vi "Read Pulse Recorder Configuration.vi"(8 "error in (no error)":errorcluster, 11 "RP Delayed in":refnum<class "RP Level.lvclass">) -> (0 "error out":errorcluster, 2 "Configuration":T1={"Pre-trigger duration"=0.01, "Post-trigger duration"=0.1, "Rate"=1000000.0, "Ranges"=[10.0], "Re-name channels"=[], "Active channels"="0:1", "External clock"=FALSE} {"Rate" format="%#_8pHz"; "Post-trigger duration" format="%#_6ps"; "Pre-trigger duration" format="%#_6ps"; "Ranges" format="%#_6pV"}, 3 "RP Delayed out":refnum<class "RP Level.lvclass">)   [LabVIEW 2018, in "RP Level.lvclass"]
uses:
  RP Level.lvclass
  NHMFL_Core/Libraries/Instruments/Pulse Driver/Pusle Driver Configuration.ctl
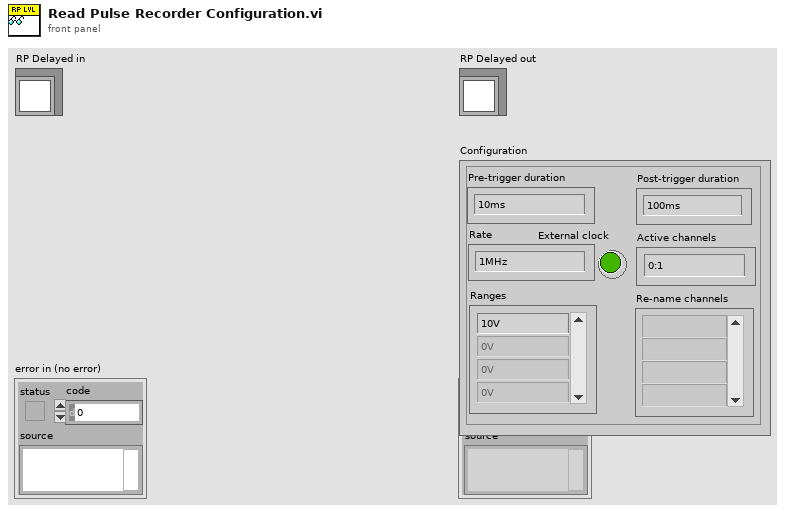
[diagram p1: front panel]
types:
  T1 = typedef "Pusle Driver Configuration.ctl" = cluster{"Pre-trigger duration":dbl, "Post-trigger duration":dbl, "Rate":dbl, "Ranges":dbl[], "Re-name channels":string[], "Active channels":string, "External clock":bool}
  T2 = typedef "RP Level Configuration.ctl" = cluster{"Pre-trigger duration":dbl, "Post-trigger duration":dbl, "Rate":dbl, "Ranges":dbl[], "Re-name channels":string[], "Active channels":string, "External clock":bool, "Output delay":dbl, "Raising edge ":bool, "Trigger level":dbl}
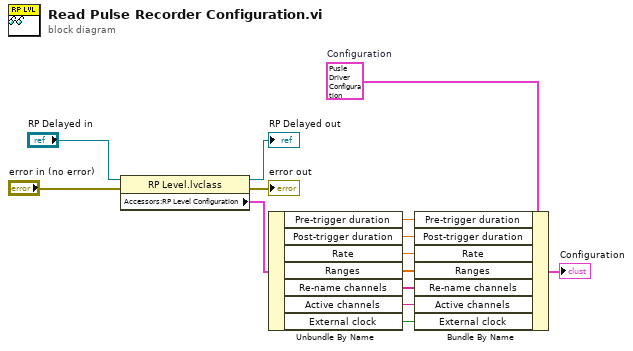
[diagram p0: block diagram]
diagram:
  w10 = T1 {"Pre-trigger duration"=0.01, "Post-trigger duration"=0.1, "Rate"=1000000.0, "Ranges"=[10.0], "Re-name channels"=[], "Active channels"="0:1", "External clock"=FALSE}  # Configuration
  n1 = property class="RP Level.lvclass"(reference="RP Delayed in", error in="error in (no error)") -> (reference out=→"RP Delayed out":refnum<class "RP Level.lvclass">, error out=→"error out":errorcluster, "Accessors:RP Level Configuration"=w9:T2)
  n2 = Unbundle By Name(w9) -> ("Pre-trigger duration"=w8:dbl, "Post-trigger duration"=w7:dbl, "Rate"=w6:dbl, "Ranges"=w5:dbl[], "Re-name channels"=w4:string[], "Active channels"=w3:string, "External clock"=w2:bool)
  n3 = Bundle By Name(cluster=w10, "Pre-trigger duration"=w8, "Post-trigger duration"=w7, "Rate"=w6, "Ranges"=w5, "Re-name channels"=w4, "Active channels"=w3, "External clock"=w2) -> (→"Configuration":T1)
